vi "Add_Next_Calib_Details.vi"(1 "% Change":dbl format="%.2f", 3 "Hours between calibrations":dbl format="%.2f", 4 "Instrument type":T1=enum."Cross wire velocity", 5 "Calib file Orig":path=path "/Hong(6%)/calib/XW Ch 1 7_10_02_5", 6 "Calib file New":path=path "/Hong(6%)/calib/XW Ch 1 7_10_02_6") -> (0 "Results Files Updated":bool)   [LabVIEW 2016]
uses:
  Controls/Cal_Inst_type.ctl
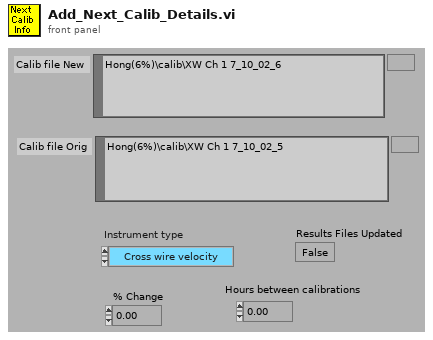
[diagram p1: front panel]
types:
  T1 = typedef "Cal_Inst_type.ctl" = enum16{"Propeller anemometer", "Pressure Transducer", "Hot wire", "Cross wire velocity", "Cross wire angle", "Generic Linear", "Generic Polynomial", "Generic BackPoly", "Fast FID", "Thermocouple", "Cold wire", "Pulsed Wire"}
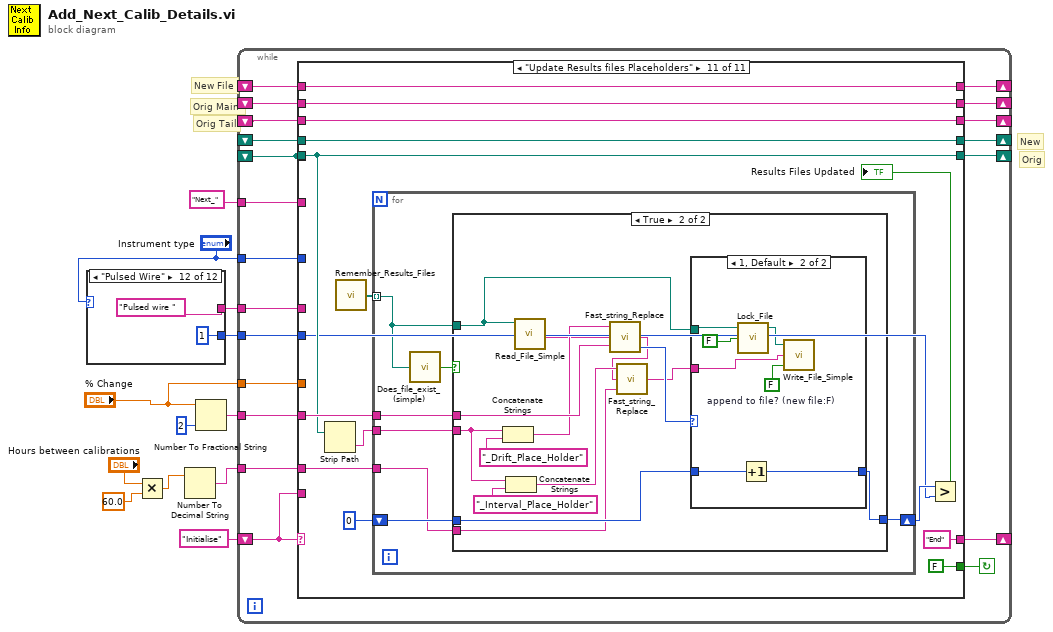
[diagram p0: block diagram]
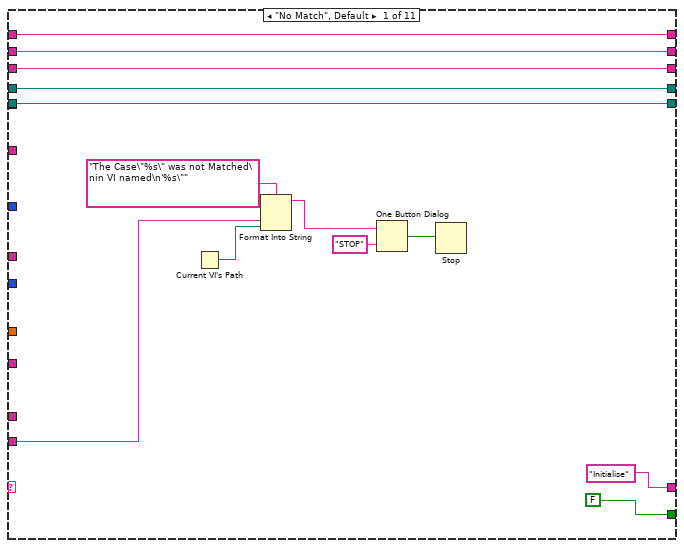
[diagram p2: hidden frame]
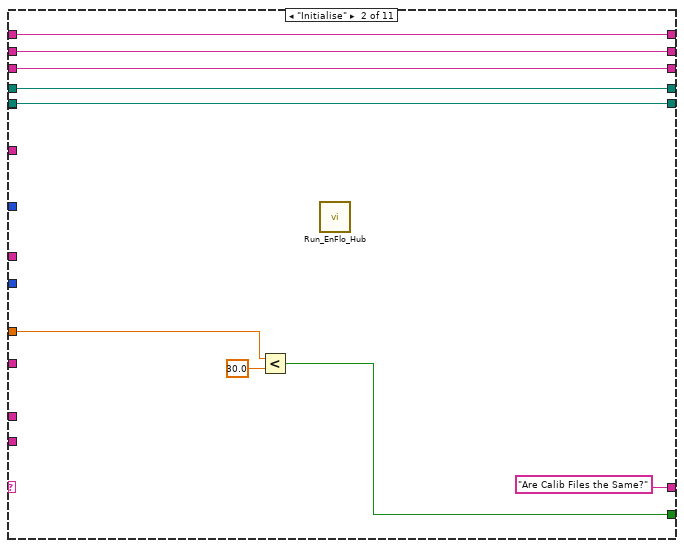
[diagram p3: hidden frame]
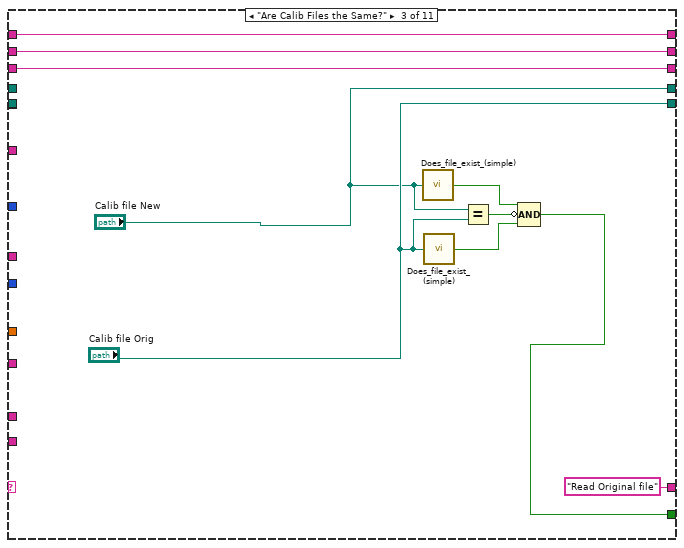
[diagram p4: hidden frame]
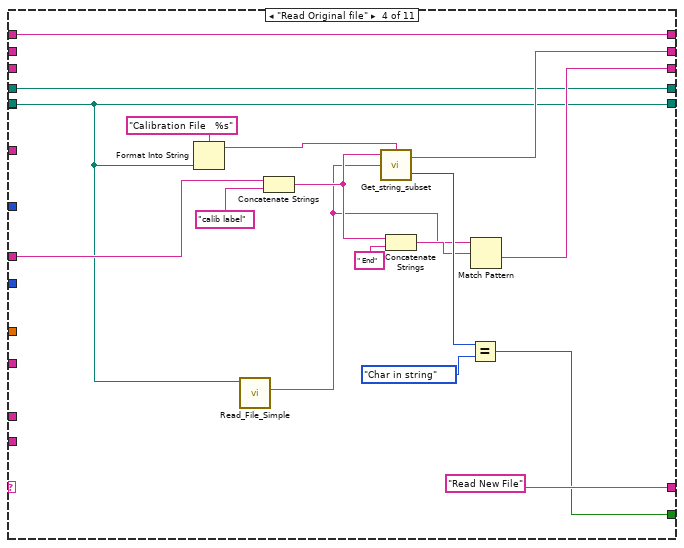
[diagram p5: hidden frame]
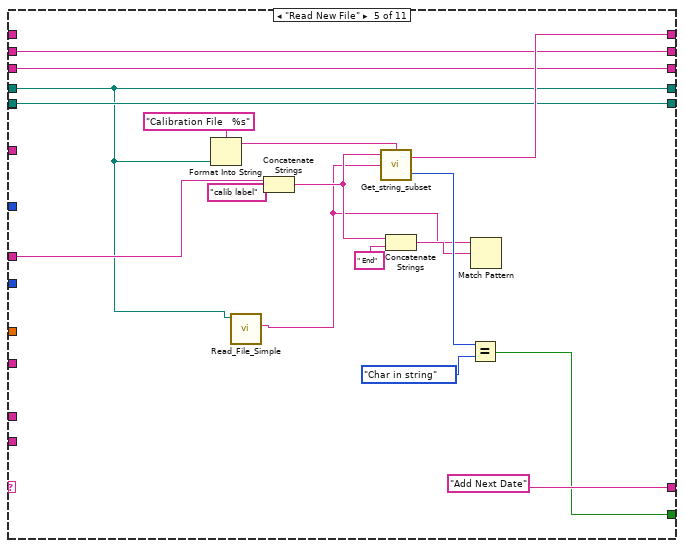
[diagram p6: hidden frame]
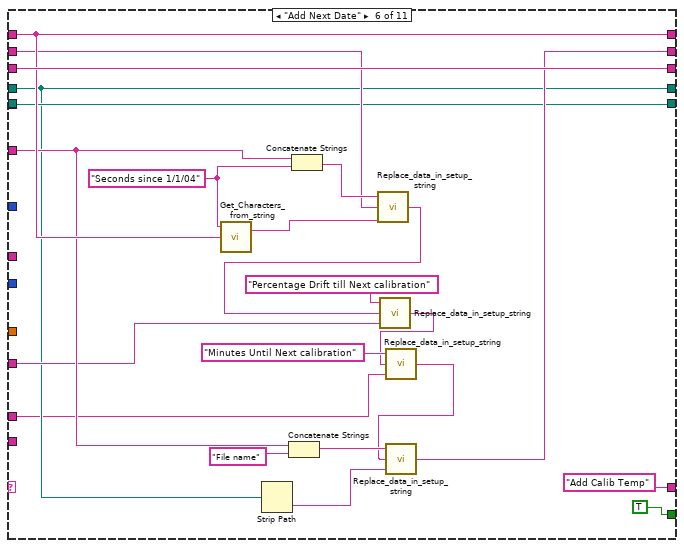
[diagram p7: hidden frame]
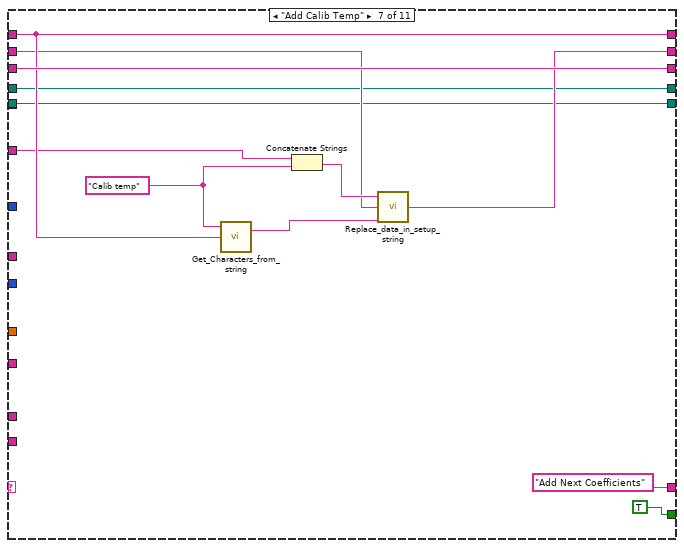
[diagram p8: hidden frame]
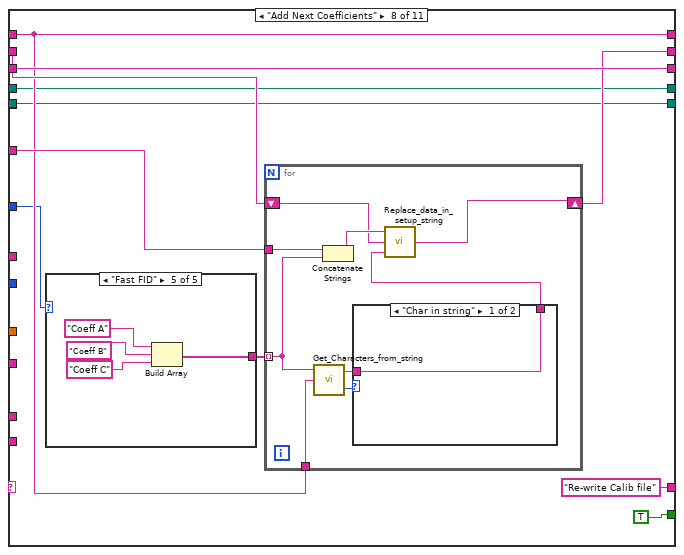
[diagram p9: hidden frame]
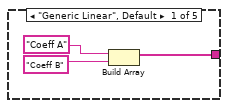
[diagram p10: hidden frame]
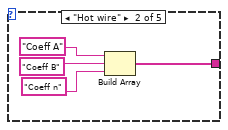
[diagram p11: hidden frame]
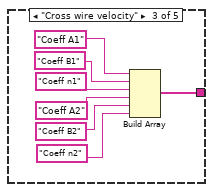
[diagram p12: hidden frame]
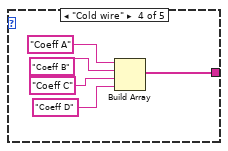
[diagram p13: hidden frame]
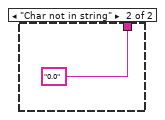
[diagram p14: hidden frame]
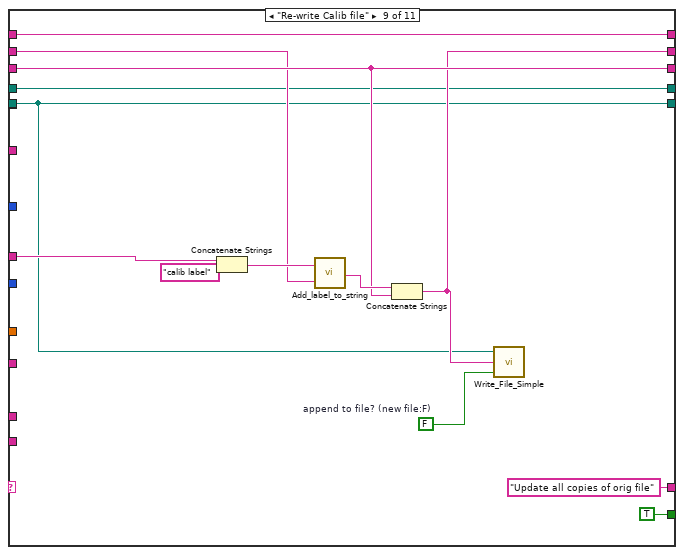
[diagram p15: hidden frame]
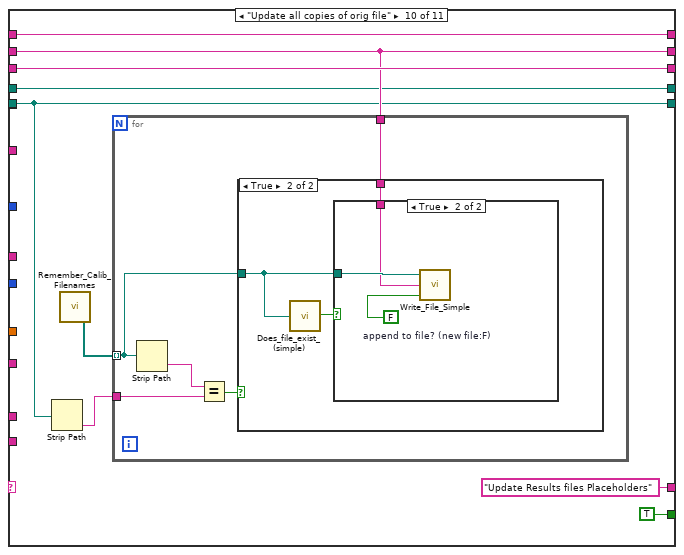
[diagram p16: hidden frame]
diagram:
  # "Orig"
  # "New"
  # "Orig Tail"
  # "New File"
  # "Orig Main"
  n1 = case shown="\"Pulsed Wire\"" "Instrument type" {
    tunnel: ["Prop " "Mano " "HW " "Cross wire velocity " "Cross wire angle " "Generic Inst " "Generic Polynomial " "Generic BackPoly " "Fast FID " "Thermocouple " "Cold wire " "Pulsed wire "] -> w10
    tunnel: [1 ("y") 1 ("y") 1 ("y") 1 ("y") 1 ("y") 1 ("y") 1 ("y") 1 ("y") 3 ("y") 1 ("y") 1 ("y") 1 ("y")] -> w2
    frame "Propeller anemometer" {
    }
    frame "Pressure Transducer" {
    }
    frame "Hot wire" {
    }
    frame "Cross wire velocity" {
    }
    frame "Cross wire angle" {
    }
    frame "Generic Linear" {
    }
    frame "Generic Polynomial" {
    }
    frame "Generic BackPoly" {
    }
    frame "Fast FID" {
    }
    frame "Thermocouple" {
    }
    frame "Cold wire" {
    }
    frame "Pulsed Wire" {
    }
  }
  n2 = Multiply(x="Hours between calibrations", y=60.0) -> (x*y=w4:dbl)
  n3 = Number To Decimal String(number=w4) -> (decimal integer string=w6:string)  [unwired: 1 out]
  n4 = Number To Fractional String(number="% Change", precision (6)=i16 2) -> (F-format string=w7:string)  [unwired: 2 out]
  n5 = while {
    shift-left: _ -> [w40]
    shift-right: [w42] -> _
    shift-left: _ -> [w43]
    shift-right: [w41] -> _
    tunnel: w7 -> [w44]
    tunnel: "Next_" -> [w45]
    tunnel: w10 -> [w46]
    shift-left: _ -> [w47]
    shift-right: [w48] -> _
    shift-left: _ -> [w49]
    shift-right: [w51] -> _
    tunnel: "Instrument type" -> [w53]
    shift-left: _ -> [w50]
    shift-right: [w52] -> _
    shift-left: "Initialise" -> [w54]
    shift-right: [w55] -> _
    tunnel: w6 -> [w39]
    tunnel: w2 -> [w38]
    tunnel: "% Change" -> [w37]
    stop <- w56 continue-if-true
    n6 = case shown="\"Update Results files Placeholders\"" w54 {
      tunnel: [FALSE w70 w81 w94 w111 TRUE TRUE TRUE TRUE TRUE FALSE] -> w56
      tunnel: ["Initialise" "Are Calib Files the Same?" "Read Original file" "Read New File" "Add Next Date" "Add Calib Temp" "Add Next Coefficients" "Re-write Calib file" "Update all copies of orig file" "Update Results files Placeholders" "End"] -> w55
      tunnel: w54 -> [w64 _ _ _ _ _ _ _ _ _ _]
      tunnel: w53 -> [_ _ _ _ _ _ _ w160 _ _ _]
      tunnel: [w61 w78 w88 w98 w120 w138 w150 w161 w212 w221 w247] -> w52
      tunnel: [w60 w76 w86 w96 w113 w139 w151 w167 w207 w220 w246] -> w51
      tunnel: w50 -> [w61 w78 w88 w98 _ w138 w150 w161 w212 w221 w247]
      tunnel: w49 -> [w60 w76 w86 _ w113 w139 w151 w167 w207 w220 w246]
      tunnel: [w59 w77 w87 w97 w114 w134 w147 w162 w204 w217 w244] -> w48
      tunnel: w47 -> [w59 w77 w87 _ w114 w137 w149 w163 w205 w217 w244]
      tunnel: w46 -> [_ _ _ w102 w117 _ _ _ w210 _ _]
      tunnel: w45 -> [_ _ _ _ _ w132 w148 w164 _ _ _]
      tunnel: w44 -> [_ _ _ _ _ w129 _ _ _ _ w242]
      tunnel: [w58 w74 "Calib file New" w93 w107 w127 w146 w158 w203 w216 w241] -> w41
      tunnel: [w57 w73 "Calib file Orig" w89 w110 w128 w145 w157 w202 w215 w240] -> w42
      tunnel: w40 -> [w57 w73 _ w89 w110 w128 w145 w157 w202 w215 _]
      tunnel: w43 -> [w58 w74 _ w93 w107 w127 w146 w158 w203 w216 w241]
      tunnel: w40 -> [_ _ _ _ _ _ _ _ _ _ w240]
      tunnel: w39 -> [_ _ _ _ _ w123 _ _ _ _ w238]
      tunnel: w38 -> [_ _ _ _ _ _ _ _ _ _ w235]
      tunnel: w37 -> [_ w72 _ _ _ _ _ _ _ _ _]
      frame "No Match", Default {
        n7 = Current VI's Path() -> (path=w63:path)
        n8 = Format Into String(format string="The Case\"%s\" was not Matched\nin VI named\n'%s\"" ("Format String"), w64, w63) -> (resulting string=w67:string)  [unwired: 2 in, 1 out]
        n9 = One Button Dialog(message=w67, button name ("OK")="STOP") -> (true=w65:bool)
        n10 = Stop(stop? (T)=w65) -> ()
      }
      frame "Initialise" {
        n11 = Less?(x=w72, y=30.0) -> (x < y?=w70:bool)
        n12 = call "Run_EnFlo_Hub.vi"() -> ()  [unwired: 1 in, 7 out]
      }
      frame "Are Calib Files the Same?" {
        n13 = call "Does_file_exist_(simple).vi"("Pathname"="Calib file New") -> ("exists?"=w83:bool)
        n14 = call "Does_file_exist_(simple).vi"("Pathname"="Calib file Orig") -> ("exists?"=w82:bool)
        n15 = Equal?(x="Calib file New", y="Calib file Orig") -> (x = y?=w84:bool)
        n16 = Compound Arithmetic op=AND(w83, invert w84, w82) -> (w81:bool)
      }
      frame "Read Original file" {
        n17 = Format Into String(format string="Calibration File   %s", w89) -> (resulting string=w90:string)  [unwired: 2 in, 1 out]
        n18 = call "Read_File_Simple.vi"("Filename"=w89) -> ("string"=w92:string)  [unwired: 2 in, 7 out]
        n19 = Concatenate Strings(w102, "calib label") -> (w99:string)
        n20 = call "Get_string_subset.vi"("String Name"=w90, "String to split"=w92, "File Label"=w99) -> ("Status"=w103:enum16{"Char in string", "Char not in string"}, "Output string"=w97:string)  [unwired: 1 in]
        n21 = Concatenate Strings(w99, " End") -> (w100:string)
        n22 = Equal?(x=w103, y=enum16{"Char in string", "Char not in string"}."Char in string" ("Status")) -> (x = y?=w94:bool)
        n23 = Match Pattern(string=w92, regular expression=w100) -> (after substring=w96:string)  [unwired: 4 out]
      }
      frame "Read New File" {
        n24 = Format Into String(format string="Calibration File   %s", w107) -> (resulting string=w106:string)  [unwired: 2 in, 1 out]
        n25 = call "Read_File_Simple.vi"("Filename"=w107) -> ("string"=w109:string)  [unwired: 2 in, 7 out]
        n26 = Concatenate Strings(w117, "calib label") -> (w112:string)
        n27 = call "Get_string_subset.vi"("String Name"=w106, "String to split"=w109, "File Label"=w112) -> ("Status"=w119:enum16{"Char in string", "Char not in string"}, "Output string"=w120:string)  [unwired: 1 in]
        n28 = Concatenate Strings(w112, " End") -> (w115:string)
        n29 = Equal?(x=w119, y=enum16{"Char in string", "Char not in string"}."Char in string" ("Status")) -> (x = y?=w111:bool)
        n30 = Match Pattern(string=w109, regular expression=w115) -> ()  [unwired: 5 out]
      }
      frame "Add Next Date" {
        w142 = "Seconds since 1/1/04"
        n31 = call "Get_Characters_from_string.vi"("Input string"=w138, "Variable name"=w142) -> ("Value"=w140:string)  [unwired: 1 in, 1 out]
        n32 = Strip Path(path=w127) -> (name=w130:string)  [unwired: 1 out]
        n33 = Concatenate Strings(w132, "File name" ("Variable name")) -> (w131:string)
        n34 = Concatenate Strings(w132, w142) -> (w141:string)
        n35 = call "Replace_data_in_setup_string.vi"("New data string"=w140, "Input string"=w137, "Variable name"=w141) -> ("Appended string"=w135:string)
        n36 = call "Replace_data_in_setup_string.vi"("New data string"=w129, "Input string"=w135, "Variable name"="Percentage Drift till Next calibration") -> ("Appended string"=w125:string)
        n37 = call "Replace_data_in_setup_string.vi"("New data string"=w123, "Input string"=w125, "Variable name"="Minutes Until Next calibration") -> ("Appended string"=w124:string)
        n38 = call "Replace_data_in_setup_string.vi"("New data string"=w130, "Input string"=w124, "Variable name"=w131) -> ("Appended string"=w134:string)
      }
      frame "Add Calib Temp" {
        w154 = "Calib temp"
        n39 = call "Get_Characters_from_string.vi"("Input string"=w150, "Variable name"=w154) -> ("Value"=w152:string)  [unwired: 1 in, 1 out]
        n40 = Concatenate Strings(w148, w154) -> (w153:string)
        n41 = call "Replace_data_in_setup_string.vi"("New data string"=w152, "Input string"=w149, "Variable name"=w153) -> ("Appended string"=w147:string)
      }
      frame "Add Next Coefficients" {
        n42 = case shown="\"Fast FID\"" w160 {
          tunnel: [w168 w171 w175 w182 w187] -> w159
          frame "Generic Linear", Default {
            n43 = Build Array("Coeff A", "Coeff B") -> (w168:string[])
          }
          frame "Hot wire" {
            n44 = Build Array("Coeff A", "Coeff B", "Coeff n") -> (w171:string[])
          }
          frame "Cross wire velocity" {
            n45 = Build Array("Coeff A1", "Coeff B1", "Coeff n1", "Coeff A2", "Coeff B2", "Coeff n2") -> (w175:string[])
          }
          frame "Cold wire" {
            n46 = Build Array("Coeff A", "Coeff B", "Coeff C", "Coeff D") -> (w182:string[])
          }
          frame "Fast FID" {
            n47 = Build Array("Coeff A", "Coeff B", "Coeff C") -> (w187:string[])
          }
        }
        n48 = for {
          tunnel: w159 -> [w198] mode=indexing
          tunnel: w164 -> [w199]
          shift-right: [w195] -> w162
          shift-left: w163 -> [w196]
          tunnel: w161 -> [w191]
          n49 = call "Get_Characters_from_string.vi"("Input string"=w191, "Variable name"=w198) -> ("Status"=w194:enum16{"Char in string", "Char not in string"}, "Value"=w193:string)  [unwired: 1 in]
          n50 = Concatenate Strings(w199, w198) -> (w197:string)
          n51 = case shown="\"Char in string\"" w194 {
            tunnel: w193 -> [w200 _]
            tunnel: [w200 "0.0"] -> w192
            frame "Char in string" {
            }
            frame "Char not in string" {
            }
          }
          n52 = call "Replace_data_in_setup_string.vi"("New data string"=w192, "Input string"=w196, "Variable name"=w197) -> ("Appended string"=w195:string)
        }
      }
      frame "Re-write Calib file" {
        w206 = FALSE  # append to file? (new file:F)
        n53 = Concatenate Strings(w210, "calib label") -> (w209:string)
        n54 = call "Add_label_to_string.vi"("String to write"=w205, "File Label"=w209) -> ("Output string"=w208:string)
        n55 = Concatenate Strings(w208, w207) -> (w204:string)
        n56 = call "Write_File_Simple.vi"("append to file? (new file:F)"=w206, "character string"=w204, "file path"=w202) -> ()  [unwired: 2 out]
      }
      frame "Update all copies of orig file" {
        n57 = Strip Path(path=w215) -> (name=w218:string)  [unwired: 1 out]
        n58 = call "Remember_Calib_Filenames.vi"() -> ("List of Filenames"=w219:path[])  [unwired: 1 in]
        n59 = for {
          tunnel: w219 -> [w225] mode=indexing
          tunnel: w218 -> [w227]
          tunnel: w217 -> [w224]
          n60 = Strip Path(path=w225) -> (name=w228:string)  [unwired: 1 out]
          n61 = Equal?(x=w228, y=w227) -> (x = y?=w226:bool)
          n62 = case shown="True" w226 {
            tunnel: w225 -> [_ w230]
            tunnel: w224 -> [_ w231]
            frame False {
            }
            frame True {
              n63 = call "Does_file_exist_(simple).vi"("Pathname"=w230) -> ("exists?"=w229:bool)
              n64 = case shown="True" w229 {
                tunnel: w230 -> [_ w233]
                tunnel: w231 -> [_ w232]
                frame False {
                }
                frame True {
                  w234 = FALSE  # append to file? (new file:F)
                  n65 = call "Write_File_Simple.vi"("append to file? (new file:F)"=w234, "character string"=w232, "file path"=w233) -> ()  [unwired: 2 out]
                }
              }
            }
          }
        }
      }
      frame "Update Results files Placeholders" {
        n66 = Strip Path(path=w240) -> (name=w243:string)  [unwired: 1 out]
        n67 = call "Remember_Results_Files.vi"() -> ("List of Filenames"=w245:path[])  [unwired: 1 in]
        n68 = for {
          tunnel: w245 -> [w254] mode=indexing
          tunnel: w243 -> [w256]
          tunnel: w242 -> [w255]
          shift-right: [w250] -> w237
          shift-left: 0 -> [w252]
          tunnel: w238 -> [w251]
          n69 = call "Does_file_exist_(simple).vi"("Pathname"=w254) -> ("exists?"=w253:bool)
          n70 = case shown="True" w253 {
            tunnel: w256 -> [_ w262]
            tunnel: w255 -> [_ w271]
            tunnel: w254 -> [_ w266]
            tunnel: [w257 w265] -> w250
            tunnel: w252 -> [w257 w264]
            tunnel: w251 -> [_ w258]
            frame False {
            }
            frame True {
              n71 = Concatenate Strings(w262, "_Drift_Place_Holder" ("Substring")) -> (w269:string)
              n72 = Concatenate Strings(w262, "_Interval_Place_Holder" ("Substring")) -> (w261:string)
              n73 = call "Read_File_Simple.vi"("Filename"=w266) -> ("string"=w268:string)  [unwired: 2 in, 7 out]
              n74 = call "Fast_string_Replace.vi"("Replace match with:"=w271, "Input String"=w268, "regular expression"=w269) -> ("Number Found"=w267:i32, "Output String"=w260:string)  [unwired: 1 out]
              n75 = call "Fast_string_Replace.vi"("Replace match with:"=w258, "Input String"=w260, "regular expression"=w261) -> ("Output String"=w259:string)  [unwired: 2 out]
              n76 = case shown="1, Default" w267 {
                tunnel: w266 -> [_ w276]
                tunnel: w259 -> [_ w273]
                tunnel: [w272 w277] -> w265
                tunnel: w264 -> [w272 w278]
                frame 0 {
                }
                frame 1, Default {
                  w279 = FALSE  # append to file? (new file:F)
                  n77 = call "Lock_File.vi"("Lock File"=FALSE, "path"=w276) -> ("dup path"=w274:path)  [unwired: 1 in, 2 out]
                  n78 = Increment(x=w278) -> (x+1=w277:i32)
                  n79 = call "Write_File_Simple.vi"("append to file? (new file:F)"=w279, "character string"=w273, "file path"=w274) -> ()  [unwired: 2 out]
                }
              }
            }
          }
        }
        n80 = Greater?(x=w237, y=w235) -> (0:→"Results Files Updated":bool)
      }
    }
  }
